vi "JobCompletionTimes.vi"() -> ()   [LabVIEW 2013]
panel:
  in  "Number Of Machines":i32=4
  in  "Number Of Jobs":i32=4
  out "Job Completion Times":i32[](array[numeric])
  in  "Gannt Chart Out":T1(array[cluster])
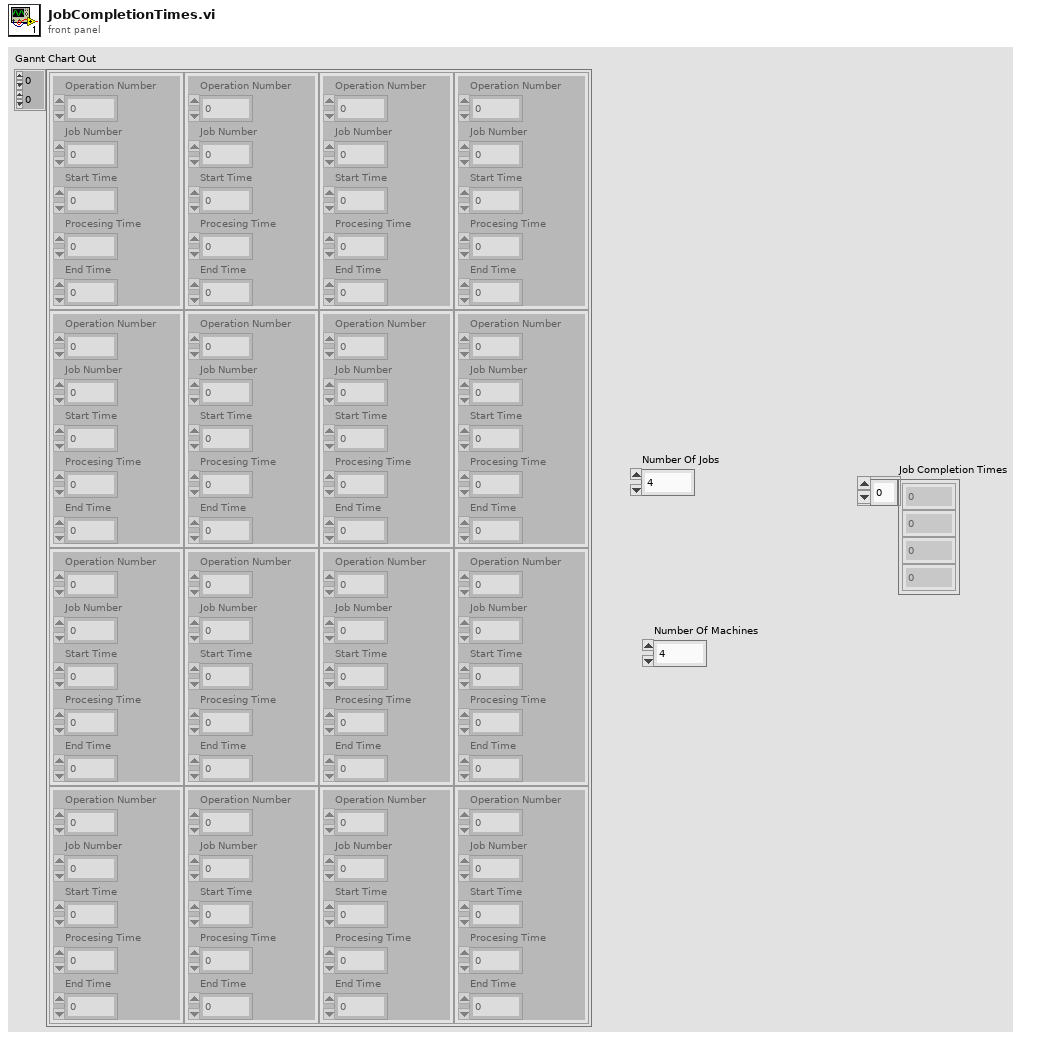
[diagram p1: front panel]
types:
  T1 = cluster{"Operation Number":i32, "Job Number":i32, "Start Time":i32, "Procesing Time":u16, "End Time":i32}[][]
  T2 = cluster{"Operation Number":i32, "Job Number":i32, "Start Time":i32, "Procesing Time":u16, "End Time":i32}[]
  T3 = cluster{"Job Number":i32, cluster{"Operation Number":i32, "Job Number":i32, "Start Time":i32, "Procesing Time":u16, "End Time":i32}}
  T4 = cluster{"Job Number":i32, cluster{"Operation Number":i32, "Job Number":i32, "Start Time":i32, "Procesing Time":u16, "End Time":i32}}[]
  T5 = cluster{"Operation Number":i32, "Job Number":i32, "Start Time":i32, "Procesing Time":u16, "End Time":i32}
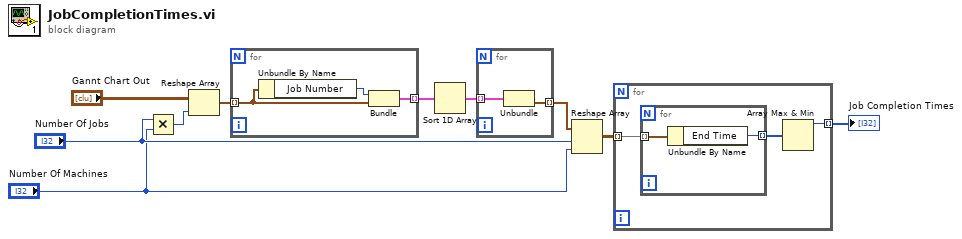
[diagram p0: block diagram]
diagram:
  n1 = Multiply(x="Number Of Jobs", y="Number Of Machines") -> (x*y=w3:i32)
  n2 = Reshape Array("Gannt Chart Out", w3) -> (w9:T2)
  n3 = for {
    tunnel: w9 -> [w12] mode=indexing
    tunnel: [w11] -> w8 mode=indexing
    n4 = Unbundle By Name(w12) -> ("Job Number"=w13:i32)
    n5 = Bundle("Job Number"=w13, w12) -> (w11:T3)  [unwired: 1 in]
  }
  n6 = Sort 1D Array(array=w8) -> (sorted array=w7:T4)
  n7 = for {
    tunnel: w7 -> [w15] mode=indexing
    tunnel: [w14] -> w6 mode=indexing
    n8 = Unbundle(w15) -> (w14:T5)  [unwired: 1 out]
  }
  n9 = Reshape Array(w6, "Number Of Jobs", "Number Of Machines") -> (w5:T1)
  n10 = for {
    tunnel: w5 -> [w18] mode=indexing
    tunnel: [w16] -> w4 mode=indexing
    n11 = for {
      tunnel: w18 -> [w20] mode=indexing
      tunnel: [w19] -> w17 mode=indexing
      n12 = Unbundle By Name(w20) -> ("End Time"=w19:i32)
    }
    n13 = Array Max & Min(array=w17) -> (max value=w16:i32)  [unwired: 3 out]
  }
  "Job Completion Times" <- w4
